vi "Clear.vi"(8 "error in (no error)":errorcluster, 11 "Result Table in":refnum<class "Result Table.lvclass">) -> (0 "error out":errorcluster, 3 "Result Table out":refnum<class "Result Table.lvclass">)   [LabVIEW 2020, in "Result Table.lvclass"]
uses:
  Result Table.lvclass
  Result Table.lvclass/Result Table.ctl
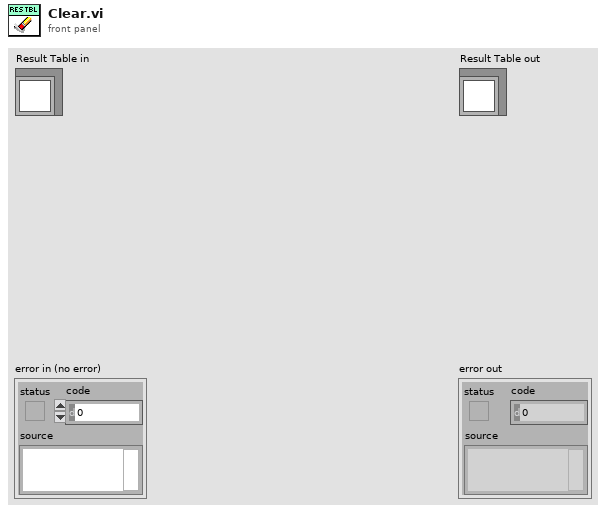
[diagram p1: front panel]
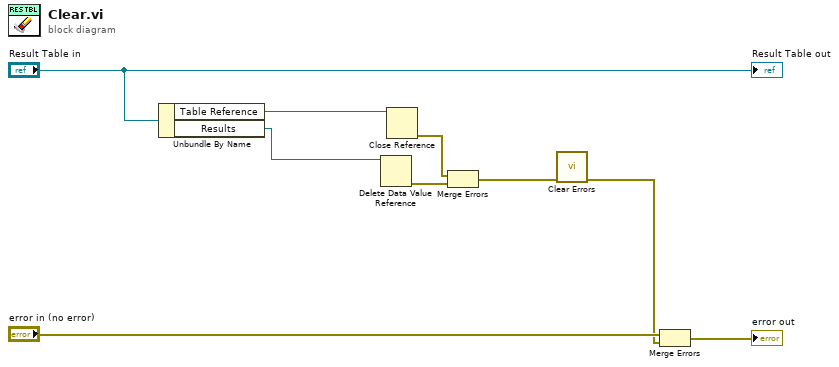
[diagram p0: block diagram]
diagram:
  n1 = Unbundle By Name("Result Table in") -> ("Table Reference"=w7:refnum<vi>, "Results"=w6:refnum<data-value>)
  n2 = Delete Data Value Reference(data value reference=w6) -> (error out=w3:errorcluster)  [unwired: 1 in, 1 out]
  n3 = Close Reference(reference=w7) -> (error out=w4:errorcluster)  [unwired: 1 in]
  n4 = Merge Errors(w4, w3) -> (w2:errorcluster)
  n5 = call <vilib>:"Clear Errors.vi"("error in (no error)"=w2) -> ("error out"=w1:errorcluster)  [unwired: 5 in, 1 out]
  n6 = Merge Errors("error in (no error)", w1) -> (→"error out":errorcluster)
  "Result Table out" <- "Result Table in"
